vi "RSNRPZ Reset.vi"(8 "error in (no error)":errorcluster, 11 "VISA session":refnum<visa-resource-name> caption="VISA resource name") -> (0 "error out":errorcluster, 3 "dup VISA session":refnum<visa-resource-name> caption="VISA resource name")   [LabVIEW 2010]
doc: "This VI resets the instrument to a known state and sends initialization commands to the instrument that set any necessary programmatic variables such as Headers Off, Short Command form, and Data Transfer Binary to the state necessary for the operation of the instrument driver."
uses:
  rsnrpz_32.dll
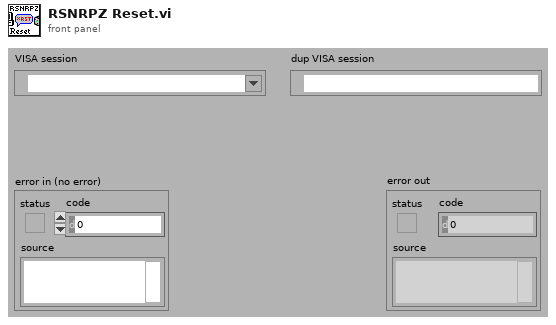
[diagram p1: front panel]
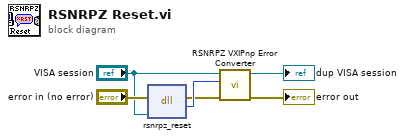
[diagram p0: block diagram]
diagram:
  n1 = dll-call lib="rsnrpz_32.dll" fn="rsnrpz_reset"(error in="error in (no error)", "VISA Session"="VISA session") -> (error out=w5:errorcluster, "Status"=w6:i32)  [unwired: 3 in, 1 out]
  n2 = call <instrlib>:"RSNRPZ VXIPnp Error Converter.vi"("error in"=w5, "VXIPnp error code"=w6, "VISA session"="VISA session") -> ("error out"=→"error out":errorcluster, "dup VISA session"=→"dup VISA session":refnum<visa-resource-name>)  [unwired: 7 in]
